vi "Lab3_3Var.vi"() -> ()   [LabVIEW 2022 SP3]
panel:
  in  "String":string
  out "Array 2":string[](array[string])
  out "Array":string[](array[string])
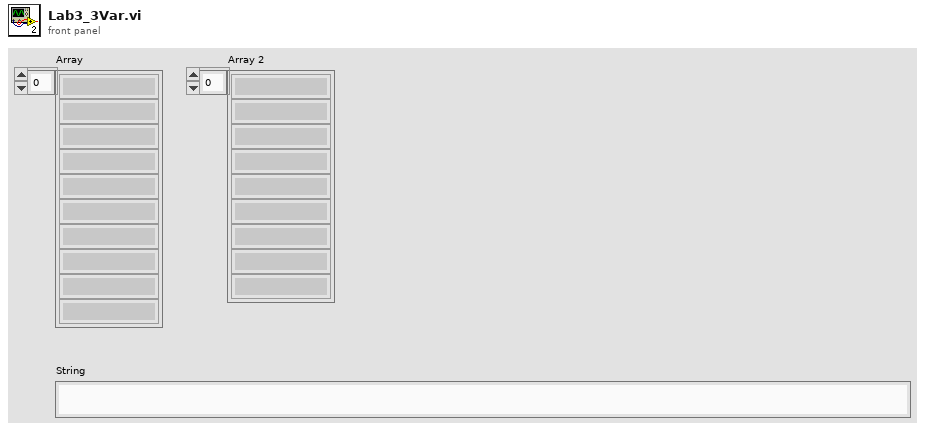
[diagram p1: front panel]
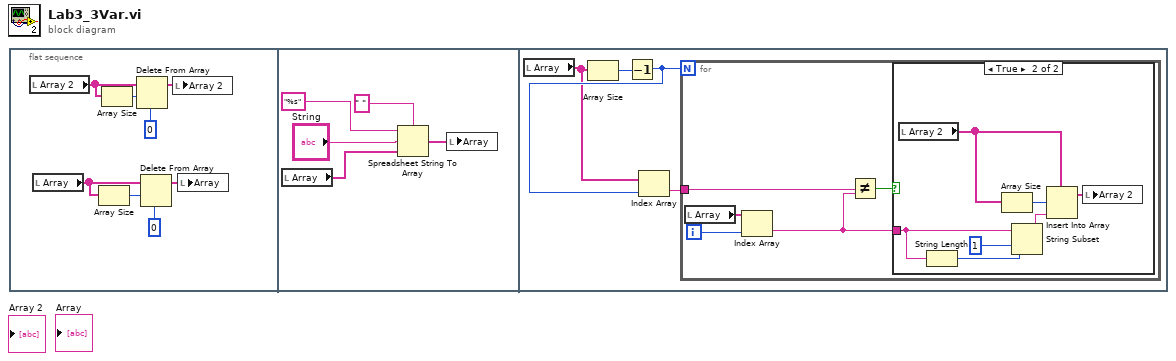
[diagram p0: block diagram]
diagram:
  n1 = flat-sequence {
    frame #0 {
      n2 = local read "Array 2"() -> (w8:string[])
      n3 = local read "Array"() -> (w3:string[])
      n4 = Array Size(array=w3) -> (size(s)=w5:i32)
      n5 = Array Size(array=w8) -> (size(s)=w7:i32)
      n6 = Delete From Array(array=w8, length=w7, index=0) -> (array with subset deleted=w2:string[])  [unwired: 1 out]
      n7 = Delete From Array(array=w3, length=w5, index=0) -> (array with subset deleted=w1:string[])  [unwired: 1 out]
      n8 = local write "Array 2"(w2) -> ()
      n9 = local write "Array"(w1) -> ()
    }
    frame #1 {
      n10 = local read "Array"() -> (w10:string[])
      n11 = Spreadsheet String To Array(delimiter (Tab)=" ", format string="%s", spreadsheet string="String", array type (2D Dbl)=w10) -> (array=w9:string[])
      n12 = local write "Array"(w9) -> ()
    }
    frame #2 {
      n13 = local read "Array"() -> (w14:string[])
      n14 = Array Size(array=w14) -> (size(s)=w17:i32)
      n15 = Decrement(x=w17) -> (x-1=w15:i32)
      n16 = Index Array(array=w14, index=w15) -> (element=w16:string)
      n17 = for {
        N: w15 -> [_]
        tunnel: w16 -> [w19]
        i -> [w21]
        n18 = local read "Array"() -> (w22:string[])
        n19 = Index Array(array=w22, index=w21) -> (element=w18:string)
        n20 = Not Equal?(x=w19, y=w18) -> (x != y?=w20:bool)
        n21 = case shown="True" w20 {
          tunnel: w18 -> [_ w23]
          frame False {
          }
          frame True {
            n22 = local read "Array 2"() -> (w28:string[])
            n23 = String Length(string=w23) -> (length=w24:i32)
            n24 = Array Size(array=w28) -> (size(s)=w29:i32)
            n25 = String Subset(string=w23, offset (0)=1, length (rest)=w24) -> (substring=w26:string)
            n26 = Insert Into Array(array=w28, index=w29, new element=w26) -> (w27:string[])
            n27 = local write "Array 2"(w27) -> ()
          }
        }
      }
    }
  }
